vi "move calculation.vi"(8 "error in (no error)":errorcluster, 10 "new Value":variant, 11 "AISAS motor in":refnum<class "AISAS motor.lvclass">) -> (0 "error out":errorcluster, 1 "Motor Direction":u8, 2 "Move param":u8[](array[numeric]), 3 "AISAS motor out":refnum<class "AISAS motor.lvclass">)   [LabVIEW 2014, in "AISAS motor.lvclass"]
uses:
  AISAS motor.lvclass
  AISAS motor.lvclass/AISAS motor.ctl
  Controls/Diffuser.ctl
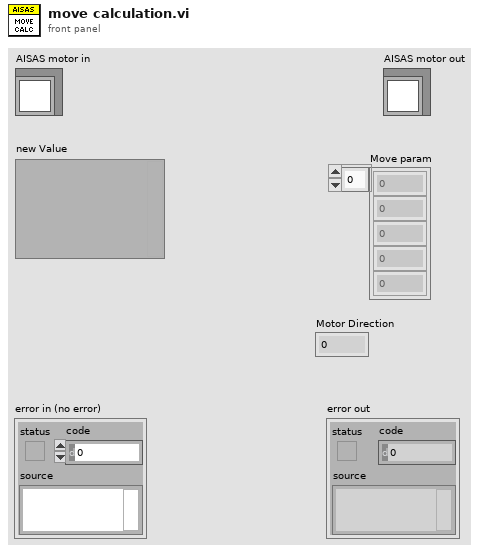
[diagram p1: front panel]
types:
  T1 = typedef "motor.ctl" = enum32{"Rotation", "Diffuser ", "Focus"}
  T2 = typedef "Diffuser.ctl" = enum16{"Out of Beam", "In Beam"}
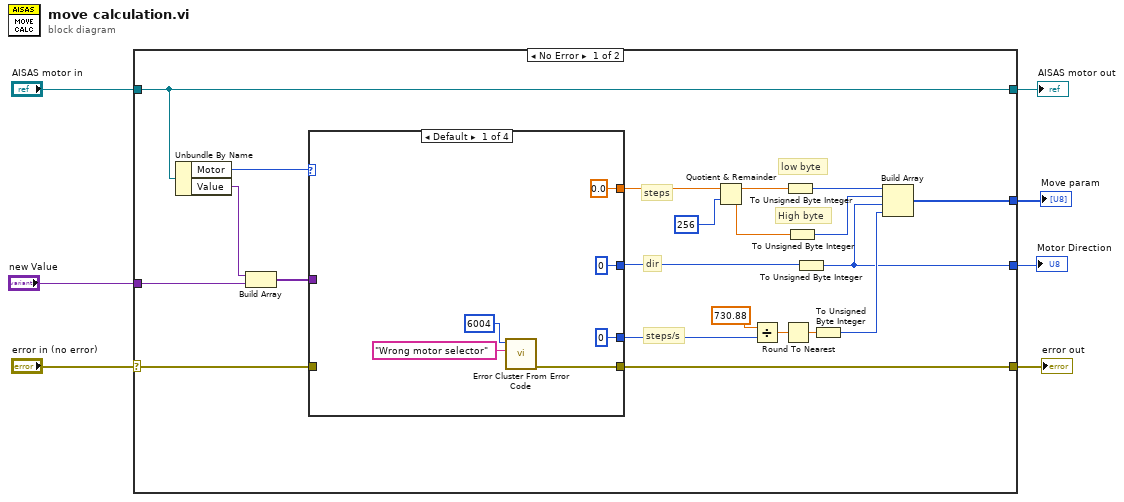
[diagram p0: block diagram]
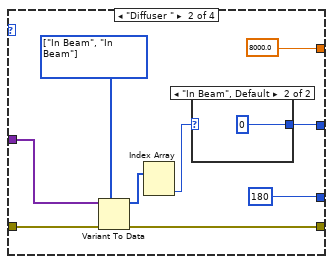
[diagram p2: hidden frame]
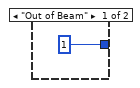
[diagram p3: hidden frame]
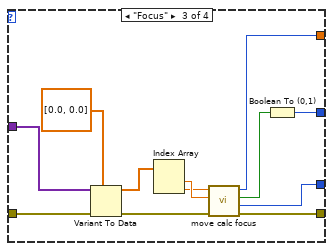
[diagram p4: hidden frame]
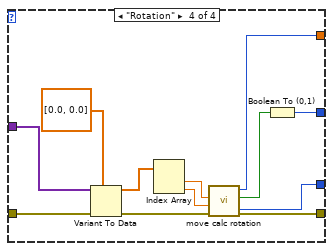
[diagram p5: hidden frame]
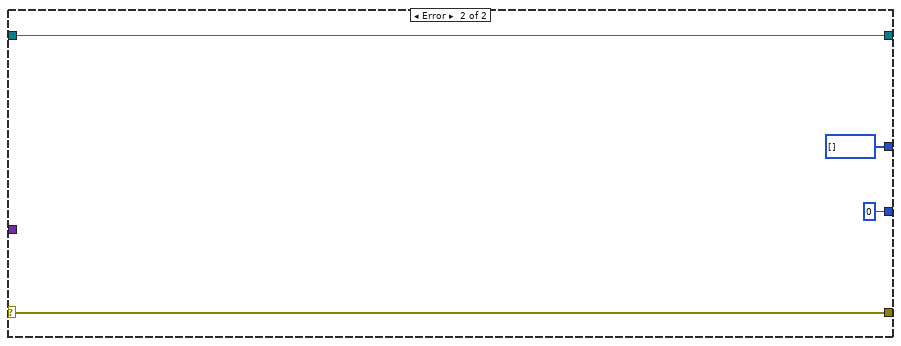
[diagram p6: hidden frame]
diagram:
  n1 = case shown="No Error" "error in (no error)" {
    selector: "error in (no error)" -> [w24 w72]
    tunnel: [w10 w72] -> w6
    tunnel: [w15 w73] -> w4
    tunnel: "AISAS motor in" -> [w15 w73]
    tunnel: "new Value" -> [w26 _]
    tunnel: [w11 u8[] []] -> w2
    tunnel: [w9 u8 0] -> w1
    frame No Error {
      # "dir"
      # "High byte"
      # "low byte"
      # "steps/s"
      # "steps"
      n2 = Unbundle By Name(w15) -> ("Motor"=w28:T1, "Value"=w27:variant)
      n3 = Build Array(w27, w26) -> (w25:variant[])
      n4 = case shown="Default" w28 {
        tunnel: w25 -> [_ w43 w57 w69]
        tunnel: w24 -> [_ w42 w56 w68]
        tunnel: [w29 w41 w53 w65] -> w10
        tunnel: [u32 0 ("steps/sec") u32 180 ("steps/sec") w48 w60] -> w20
        tunnel: [0.0 ("Steps") 8000.0 ("Steps") w49 w61] -> w16
        tunnel: [i16 0 w35 w46 w58] -> w8
        frame Default {
          n5 = call <vilib>:"Error Cluster From Error Code.vi"("error message (\"\")"="Wrong motor selector" ("error message (\"\")"), "error code (0)"=6004) -> ("error out"=w29:errorcluster)  [unwired: 7 in]
        }
        frame "Diffuser " {
          w37 = T2[] [enum."In Beam", enum."In Beam"] items=["Out of Beam", "In Beam"]
          n6 = Variant To Data(error in=w42, type=w37, Variant=w43) -> (data=w40:T2[], error out=w41:errorcluster)
          n7 = Index Array(array=w40) -> (element #2=w36:T2)  [unwired: 2 in, 1 out]
          n8 = case shown="\"In Beam\", Default" w36 {
            tunnel: [i16 1 i16 0] -> w35
            frame "Out of Beam" {
            }
            frame "In Beam", Default {
            }
          }
        }
        frame "Focus" {
          n9 = Variant To Data(error in=w56, type=dbl[] [0.0, 0.0], Variant=w57) -> (data=w52:dbl[], error out=w54:errorcluster)
          n10 = Index Array(array=w52) -> (element #1=w51:dbl, element #2=w50:dbl)  [unwired: 2 in]
          n11 = call "move calc focus.vi"("error in (no error)"=w54, "old Focus"=w51, "new Focus"=w50) -> ("error out"=w53:errorcluster, "Velocity"=w48:i32, "Motor Direction"=w47:bool, "Steps"=w49:i32)  [unwired: 4 in]
          n12 = Boolean To (0,1)(Boolean=w47) -> (0, 1=w46:i16)
        }
        frame "Rotation" {
          n13 = Variant To Data(error in=w68, type=dbl[] [0.0, 0.0], Variant=w69) -> (data=w64:dbl[], error out=w66:errorcluster)
          n14 = Index Array(array=w64) -> (element #1=w63:dbl, element #2=w62:dbl)  [unwired: 2 in]
          n15 = call "move calc rotation.vi"("error in (no error)"=w66, "New Value"=w62, "Old Value"=w63) -> ("error out"=w65:errorcluster, "Direction"=w59:bool, "steps"=w61:i32, "Degrees"=w60:i32)  [unwired: 4 in, 1 out]
          n16 = Boolean To (0,1)(Boolean=w59) -> (0, 1=w58:i16)
        }
      }
      n17 = Quotient & Remainder(x=w16, y=256) -> (x-y*floor(x/y)=w17:dbl, floor(x/y)=w18:dbl)
      n18 = Divide(x=730.88, y=w20) -> (x/y=w23:dbl)
      n19 = Round To Nearest(number=w23) -> (nearest integer value=w22:dbl)
      n20 = To Unsigned Byte Integer(number=w17) -> (unsigned 8bit integer=w14:u8)
      n21 = To Unsigned Byte Integer(number=w18) -> (unsigned 8bit integer=w12:u8)
      n22 = To Unsigned Byte Integer(number=w8) -> (unsigned 8bit integer=w9:u8)
      n23 = To Unsigned Byte Integer(number=w22) -> (unsigned 8bit integer=w13:u8)
      n24 = Build Array(w14, w12, w9, w13) -> (w11:u8[])
    }
    frame Error {
    }
  }
  "error out" <- w6
  "AISAS motor out" <- w4
  "Move param" <- w2
  "Motor Direction" <- w1
